vi "Disable Type Items.vi"(8 "error in (no error)":errorcluster, 11 "Numeric Data Type in":refnum<class "Numeric Data Type.lvclass">) -> (0 "error out":errorcluster, 3 "Numeric Data Type out":refnum<class "Numeric Data Type.lvclass">)   [LabVIEW 2018, in "Numeric Data Type.lvclass"]
uses:
  Numeric Data Type.lvclass
  Numeric Data Type.lvclass/Numeric Data Type.ctl
  Numeric Format Enum.ctl
  Reference Display Type.vi
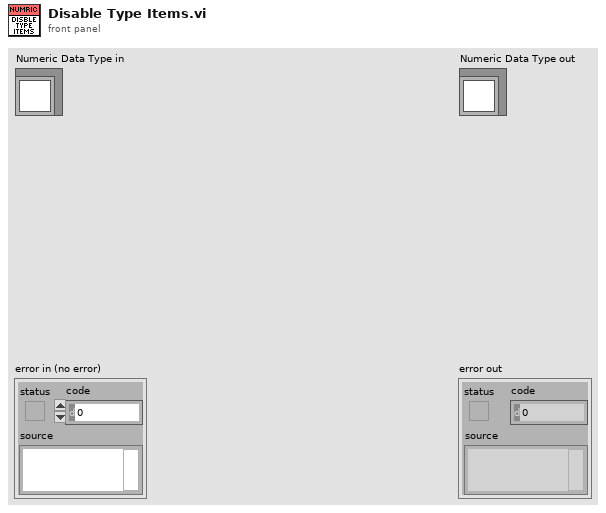
[diagram p1: front panel]
types:
  T1 = typedef "Numeric Data Type.lvclass/Numeric Format Enum.ctl" = enum16{"Floating Point Notation", "Scientific Notation", "Engineering Notation", "SI Notation", "<not used>", "Decimal", "Hexadecimal", "Octal", "Binary", "<not used 2>", "Absolute Time", "Relative Time"}
  T2 = typedef "Numeric Data Type.lvclass/Representation Enum.ctl" = enum16{"Extended (EXT)", "Double (DBL)", "Single (SGL)", "Fixed-Point (FXP)", "Quad Integer (I64)", "Long Integer (I32)", "Word Integer (I16)", "Byte Integer (I8)", "Unsigned Quad (U64)", "Unsigned Long (U32)", "Unsigned Word (U16)", "Unsigned Byte (U8)", "Complex Extended (CXT)", "Complex Double (CDB)", "Complex Single (CSG)"}
  T3 = typedef "Numeric Data Type.lvclass/Numeric Info.ctl" = cluster{"Minimum Field Width":i32, "Digits of Precision":i32, "Numeric Format":T1, "Precision Type":T4, "Hide trailing zeros":bool, "exponent":bool, "just/pad":T5, "Modifiers":string}
  T4 = typedef "Numeric Data Type.lvclass/Precision Type.ctl" = enum16{"Digits of precision", "Significant digits"}
  T5 = typedef "Numeric Data Type.lvclass/Padding.ctl" = enum16{"Pad with spaces on left", "Pad with spaces on right", "Pad with zeros on left"}
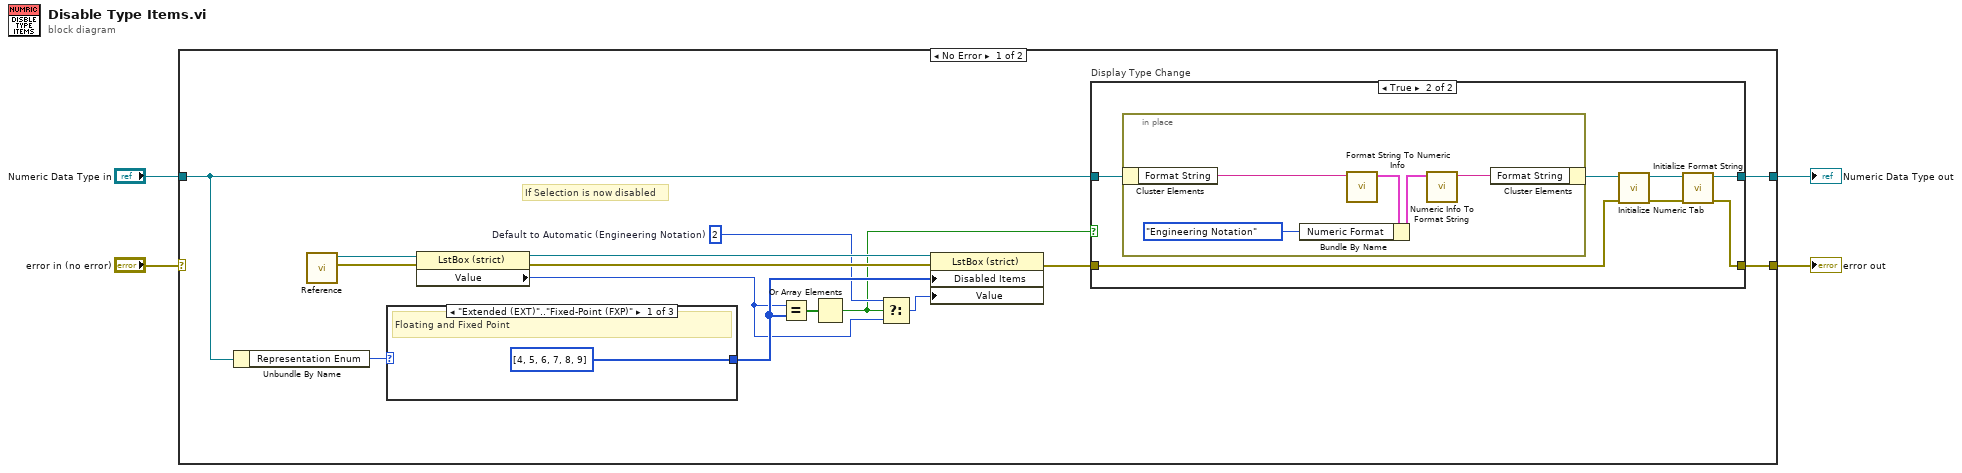
[diagram p0: block diagram]
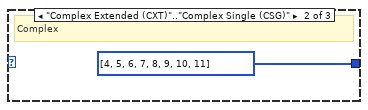
[diagram p3: hidden frame]
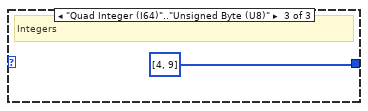
[diagram p4: hidden frame]
diagram:
  n1 = case shown="No Error" "error in (no error)" {
    selector: "error in (no error)" -> [_ w38]
    tunnel: [w6 w38] -> w3
    tunnel: [w7 w37] -> w1
    tunnel: "Numeric Data Type in" -> [w8 w37]
    frame No Error {
      w12 = 2  # Default to Automatic (Engineering Notation)
      # "If Selection is now disabled"
      n2 = Unbundle By Name(w8) -> ("Representation Enum"=w5:T2)
      n3 = call-poly "Reference.vi"() -> ("error out"=w19:errorcluster, "Display Type"=w17:refnum<vi>)  [unwired: 10 in]
      n4 = case shown="\"Extended (EXT)\"..\"Fixed-Point (FXP)\"" w5 {
        tunnel: [i32[] [4, 5, 6, 7, 8, 9] i32[] [4, 5, 6, 7, 8, 9, 10, 11] i32[] [4, 9]] -> w15
        frame "Extended (EXT)".."Fixed-Point (FXP)" {
          # "Floating and Fixed Point"
        }
        frame "Complex Extended (CXT)".."Complex Single (CSG)" {
          # "Complex"
        }
        frame "Quad Integer (I64)".."Unsigned Byte (U8)" {
          # "Integers"
        }
      }
      n5 = property class="LstBox (strict)"(reference=w17, error in=w19) -> (reference out=w16:refnum<vi>, error out=w18:errorcluster, "Value"=w13:i32)
      n6 = Equal?(x=w13, y=w15) -> (x = y?=w14:bool[])
      n7 = Or Array Elements(Boolean array=w14) -> (logical OR=w10:bool)
      n8 = Select(t=w12, s=w10, f=w13) -> (s? t:f=w11:i32)
      n9 = property on="Property Node" class="LstBox (strict)"(reference=w16, error in=w18, "Disabled Items"=w15, "Value"=w11) -> (error out=w9:errorcluster)  [unwired: 1 out]
      n10 = case "Display Type Change" shown="True" w10 {
        tunnel: w9 -> [w20 w23]
        tunnel: w8 -> [w21 w28]
        tunnel: [w21 w25] -> w7
        tunnel: [w20 w22] -> w6
        frame False {
        }
        frame True {
          n11 = in-place {
            n12 = in-place-cluster #1(w28) -> ("Format String"=w33:string)
            n13 = call "Format String To Numeric Info.vi"("Format String"=w33) -> ("Numeric Format & Precision Info"=w32:T3)  [unwired: 10 in]
            n14 = Bundle By Name(cluster=w32, "Numeric Format"=Numeric_Format_Enum."Engineering Notation") -> (w30:T3)
            n15 = call "Numeric Info To Format String.vi"("Numeric Format & Precision Info"=w30) -> ("Format String"=w29:string)  [unwired: 10 in]
            n16 = in-place-cluster #1("Format String"=w29) -> (w27:refnum<class "Numeric Data Type.lvclass">)
          }
          n17 = call "Initialize Numeric Tab.vi"("error in (no error)"=w23, "Numeric Data Type in"=w27) -> ("error out"=w24:errorcluster, "Numeric Data Type (dub)"=w26:refnum<class "Numeric Data Type.lvclass">)  [unwired: 8 in]
          n18 = call "Initialize Format String.vi"("error in (no error)"=w24, "Numeric Data Type in"=w26) -> ("error out"=w22:errorcluster, "Numeric Data Type (dup)"=w25:refnum<class "Numeric Data Type.lvclass">)  [unwired: 8 in]
        }
      }
    }
    frame Error {
    }
  }
  "error out" <- w3
  "Numeric Data Type out" <- w1
